vi "Pre Launch Init.vi"(11 "RootActor in":refnum<class "RootActor.lvclass">) -> (0 "error out":errorcluster, 3 "RootActor out":refnum<class "RootActor.lvclass">)   [LabVIEW 2020, in "RootActor.lvlib" / "RootActor.lvclass"]
doc: "(<B>Filename</B>: Actor Framework.lvlib:Actor.lvclass:Pre Launch Init.vi)\n\nDefines behavior that occurs after the Launch Nested Actor method is invoked but before the actor's Actor Core method begins running.\n\nBy default, this method does nothing. A descendant class may override it to define behavior."
uses:
  RootActor.lvclass
  RootActor.lvclass/RootActor.ctl
  <vilib>/ActorFramework/Actor/Actor.lvclass
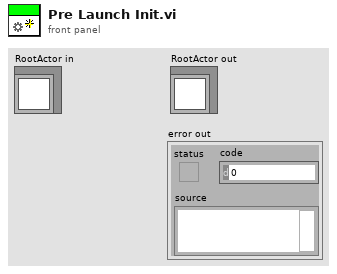
[diagram p1: front panel]
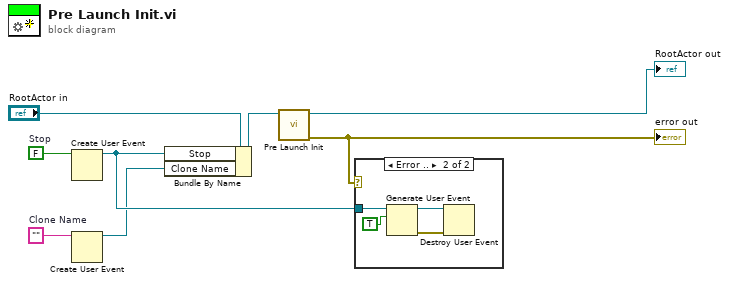
[diagram p0: block diagram]
diagram:
  w3 = ""  # Clone Name
  w7 = FALSE  # Stop
  n1 = Create User Event(user event datatype=w7) -> (user event=w2:refnum<user-event>)  [unwired: 1 in, 1 out]
  n2 = Create User Event(user event datatype=w3) -> (user event=w1:refnum<user-event>)  [unwired: 1 in, 1 out]
  n3 = Bundle By Name(cluster="RootActor in", "Stop"=w2, "Clone Name"=w1) -> (w4:refnum<class "RootActor.lvclass">)
  n4 = call-parent "Pre Launch Init.vi"("Actor in"=w4) -> ("error out"=w6:errorcluster, "Actor out"=→"RootActor out":refnum<class "RootActor.lvclass">)  [unwired: 9 in]
  "error out" <- w6
  n5 = case shown="Error .." w6 {
    tunnel: w2 -> [_ w12]
    frame No Error {
    }
    frame Error {
      n6 = Generate User Event(user event=w12, event data cluster=TRUE ("event data")) -> (user event out=w9:refnum<user-event>, error out=w10:errorcluster)  [unwired: 2 in]
      n7 = Destroy User Event(user event=w9, error in=w10) -> ()  [unwired: 1 out]
    }
  }
